vi "SLM Standard Messenger.vi"(0 "Notifier Name":string, 1 "Flat On/Off":bool, 2 "Vortex On/Off":bool, 3 "Top Hat On/Off":bool, 4 "Top Hat Radius":dbl, 5 "Mode Amounts":dbl[](array[numeric]), 6 "Holo Size (px)":i32, 7 "Number of Modes":i32, 8 "SLM Actions":T2, 9 "Holo Position":i32[](array[numeric])) -> (14 "Notifier Name Dup":string, 17 "SLM Status":T1)   [LabVIEW 2018]
uses:
  X10468 Series/X10468 Controls/X10468 SLM Actions.ctl
  X10468 Series/X10468 Controls/X10468 SLM Notifier.ctl
  <vilib>/vision/Image Controls.llb/IMAQ Image.ctl
panel:
  out "Error":errorcluster
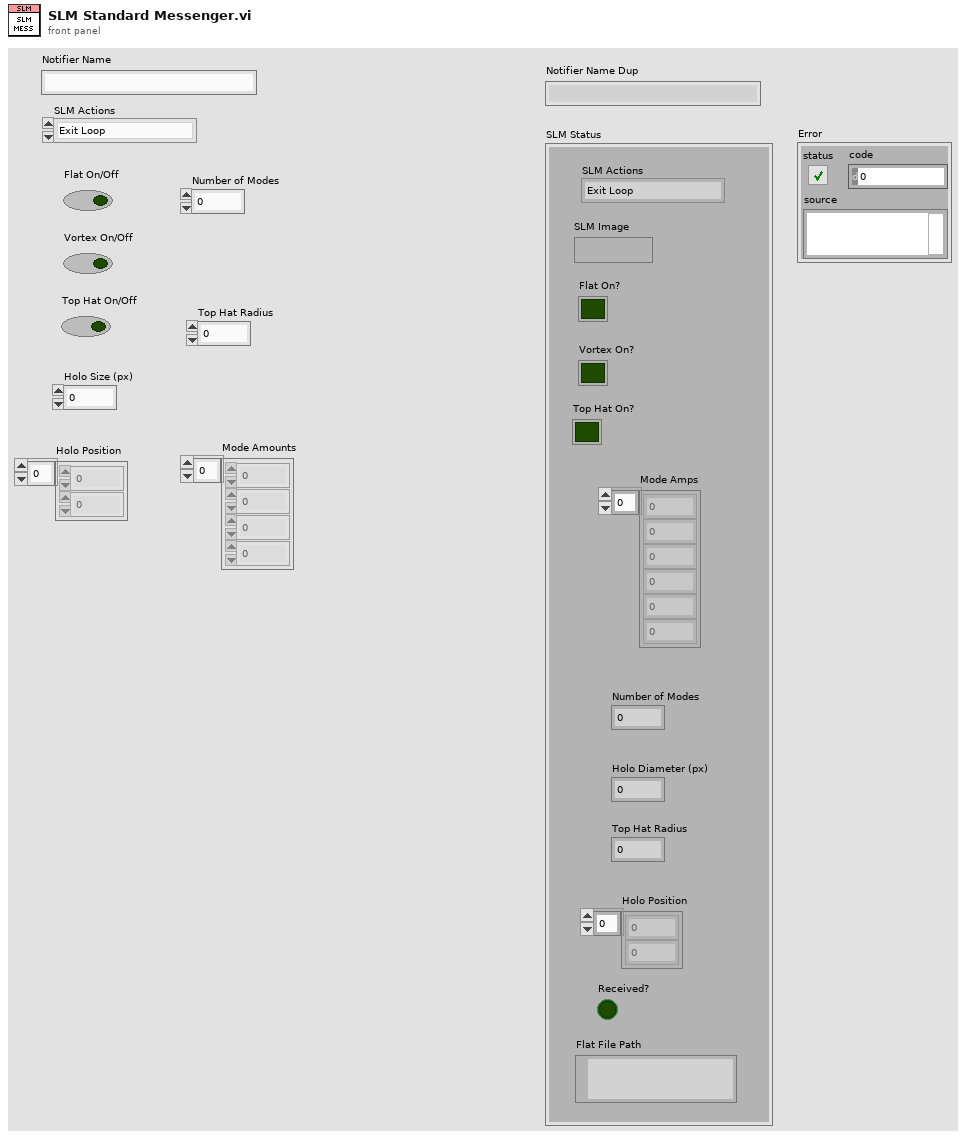
[diagram p1: front panel]
types:
  T1 = typedef "X10468 SLM Notifier.ctl" = cluster{"SLM Actions":T2, "SLM Image":T3, "Flat On?":bool, "Vortex On?":bool, "Top Hat On?":bool, "Mode Amps":dbl[], "Number of Modes":i32, "Holo Diameter (px)":i32, "Top Hat Radius":dbl, "Holo Position":i32[], "Received?":bool, "Flat File Path":path}
  T2 = typedef "X10468 SLM Actions.ctl" = enum16{"Exit Loop", "Get Settings", "Set Flat File", "Change Holo Size", "Change Num Modes", "Change Holo Position", "Change Top Hat Size", "Change Vortex Direction", "Change Mode Amounts", "Flat On/Off", "Vortex On/Off", "Top Hat On/Off", "Make Hologram", "Update SLM Display", "Quit"}
  T3 = typedef "IMAQ Image.ctl" = refnum<image>
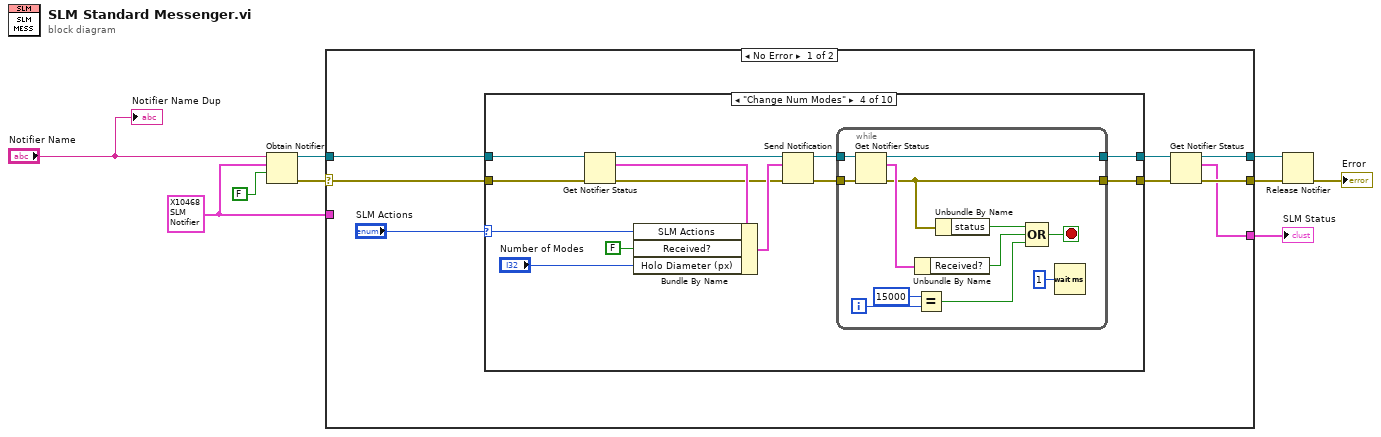
[diagram p0: block diagram]
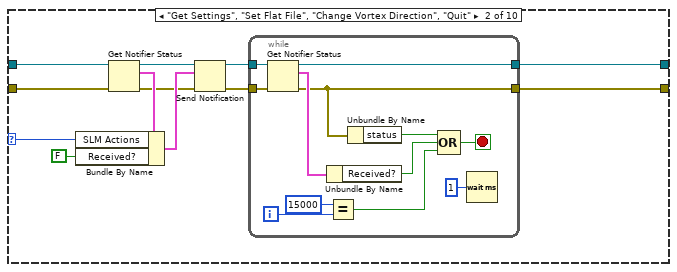
[diagram p3: hidden frame]
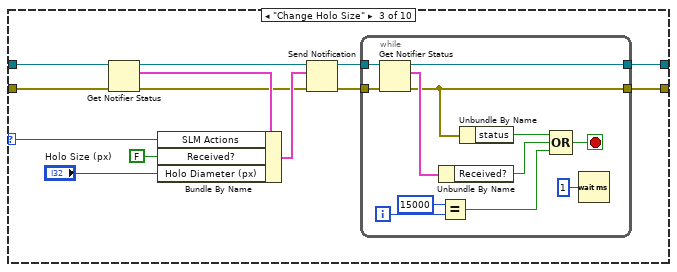
[diagram p4: hidden frame]
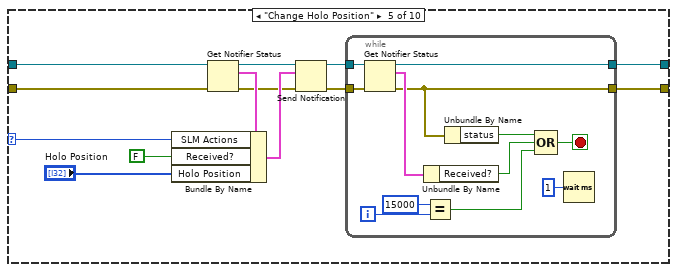
[diagram p5: hidden frame]
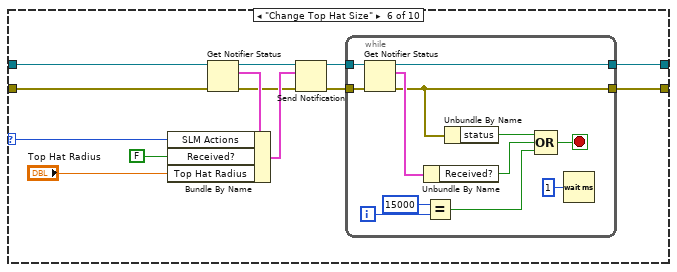
[diagram p6: hidden frame]
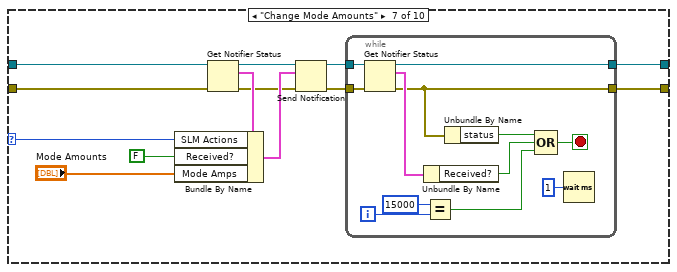
[diagram p7: hidden frame]
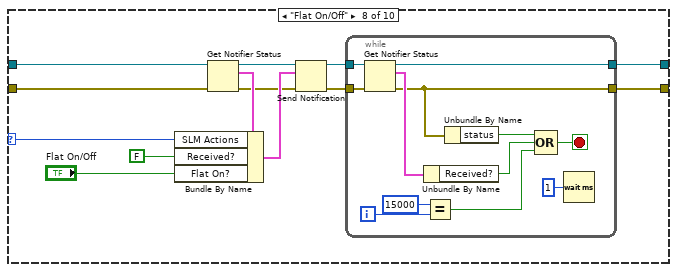
[diagram p8: hidden frame]
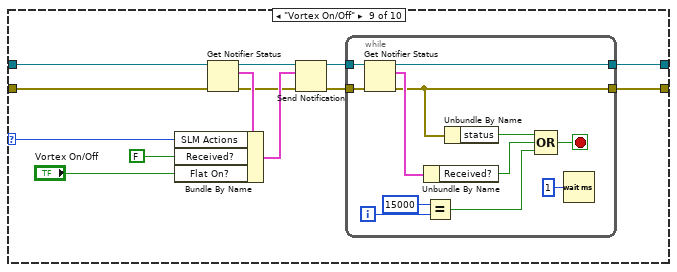
[diagram p9: hidden frame]
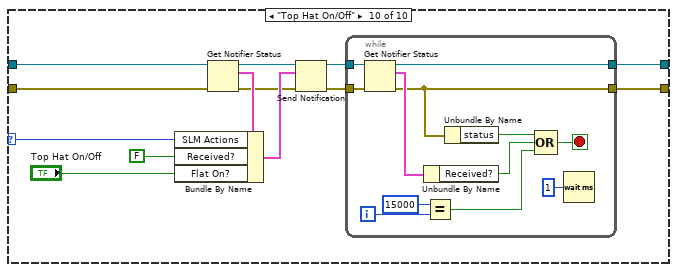
[diagram p10: hidden frame]
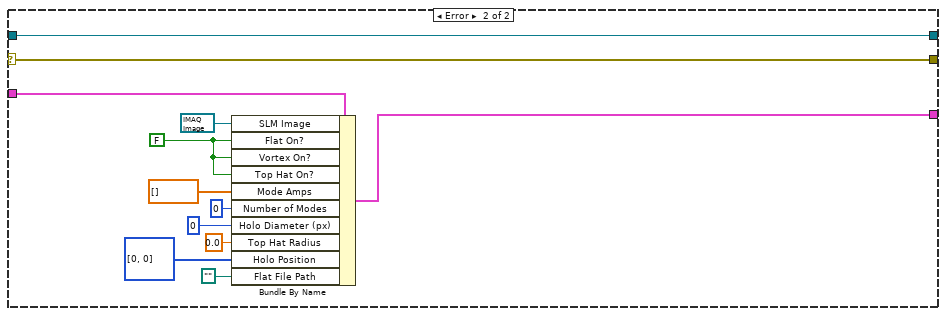
[diagram p11: hidden frame]
diagram:
  w1 = T1 {"SLM Actions"=enum."Exit Loop", "SLM Image"=refnum, "Flat On?"=FALSE, "Vortex On?"=FALSE, "Top Hat On?"=FALSE, "Mode Amps"=[], "Number of Modes"=0, "Holo Diameter (px)"=0, "Top Hat Radius"=0.0, "Holo Position"=[], "Received?"=FALSE, "Flat File Path"=path ""} ("SLM Notifier")
  n1 = Obtain Notifier(name (unnamed)="Notifier Name", notification data type=w1, create if not found? (T)=FALSE) -> (notifier out=w7:refnum<notifier>, error out=w6:errorcluster)  [unwired: 1 in, 1 out]
  n2 = case shown="No Error" w6 {
    selector: w6 -> [w15 w254]
    tunnel: w7 -> [w16 w255]
    tunnel: [w12 w255] -> w5
    tunnel: [w11 w254] -> w4
    tunnel: [w10 w252] -> w2
    tunnel: w1 -> [_ w253]
    frame No Error {
      n3 = case shown="\"Change Num Modes\"" "SLM Actions" {
        selector: "SLM Actions" -> [_ w28 w53 w78 w103 w128 w153 w178 w203 w228]
        tunnel: w16 -> [w19 w31 w56 w81 w106 w131 w156 w181 w206 w231]
        tunnel: w15 -> [w18 w26 w51 w76 w101 w126 w151 w176 w201 w226]
        tunnel: [w19 w21 w46 w71 w96 w121 w146 w171 w196 w221] -> w14
        tunnel: [w18 w20 w45 w70 w95 w120 w145 w170 w195 w220] -> w13
        frame "Exit Loop", Default {
        }
        frame "Get Settings", "Set Flat File", "Change Vortex Direction", "Quit" {
          n4 = Get Notifier Status(notifier=w31, error in (no error)=w26) -> (notifier out=w30:refnum<notifier>, current notification=w29:T1, error out=w25:errorcluster)  [unwired: 2 out]
          n5 = Bundle By Name(cluster=w29, "SLM Actions"=w28, "Received?"=FALSE) -> (w27:T1)
          n6 = Send Notification(notification=w27, notifier=w30, error in (no error)=w25) -> (notifier out=w23:refnum<notifier>, error out=w22:errorcluster)
          n7 = while {
            tunnel: w23 -> [w43]
            tunnel: [w40] -> w21
            tunnel: w22 -> [w37]
            tunnel: [w36] -> w20
            i -> [w39]
            stop <- w32 stop-if-true
            n8 = Get Notifier Status(notifier=w43, error in (no error)=w37) -> (notifier out=w40:refnum<notifier>, current notification=w42:T1, error out=w36:errorcluster)  [unwired: 2 out]
            n9 = Unbundle By Name(w42) -> ("Received?"=w34:bool)
            n10 = Equal?(x=15000, y=w39) -> (x = y?=w33:bool)
            n11 = Unbundle By Name(w36) -> ("status"=w35:bool)
            n12 = Compound Arithmetic op=OR(w35, w34, w33) -> (w32:bool)
            n13 = Wait (ms)(milliseconds to wait=u32 1) -> ()  [unwired: 1 out]
          }
        }
        frame "Change Holo Size" {
          n14 = Get Notifier Status(notifier=w56, error in (no error)=w51) -> (notifier out=w55:refnum<notifier>, current notification=w54:T1, error out=w50:errorcluster)  [unwired: 2 out]
          n15 = Bundle By Name(cluster=w54, "SLM Actions"=w53, "Received?"=FALSE, "Holo Diameter (px)"="Holo Size (px)") -> (w52:T1)
          n16 = Send Notification(notification=w52, notifier=w55, error in (no error)=w50) -> (notifier out=w48:refnum<notifier>, error out=w47:errorcluster)
          n17 = while {
            tunnel: w48 -> [w68]
            tunnel: [w65] -> w46
            tunnel: w47 -> [w62]
            tunnel: [w61] -> w45
            i -> [w64]
            stop <- w57 stop-if-true
            n18 = Get Notifier Status(notifier=w68, error in (no error)=w62) -> (notifier out=w65:refnum<notifier>, current notification=w67:T1, error out=w61:errorcluster)  [unwired: 2 out]
            n19 = Unbundle By Name(w67) -> ("Received?"=w59:bool)
            n20 = Equal?(x=15000, y=w64) -> (x = y?=w58:bool)
            n21 = Unbundle By Name(w61) -> ("status"=w60:bool)
            n22 = Compound Arithmetic op=OR(w60, w59, w58) -> (w57:bool)
            n23 = Wait (ms)(milliseconds to wait=u32 1) -> ()  [unwired: 1 out]
          }
        }
        frame "Change Num Modes" {
          n24 = Get Notifier Status(notifier=w81, error in (no error)=w76) -> (notifier out=w80:refnum<notifier>, current notification=w79:T1, error out=w75:errorcluster)  [unwired: 2 out]
          n25 = Bundle By Name(cluster=w79, "SLM Actions"=w78, "Received?"=FALSE, "Holo Diameter (px)"="Number of Modes") -> (w77:T1)
          n26 = Send Notification(notification=w77, notifier=w80, error in (no error)=w75) -> (notifier out=w73:refnum<notifier>, error out=w72:errorcluster)
          n27 = while {
            tunnel: w73 -> [w93]
            tunnel: [w90] -> w71
            tunnel: w72 -> [w87]
            tunnel: [w86] -> w70
            i -> [w89]
            stop <- w82 stop-if-true
            n28 = Get Notifier Status(notifier=w93, error in (no error)=w87) -> (notifier out=w90:refnum<notifier>, current notification=w92:T1, error out=w86:errorcluster)  [unwired: 2 out]
            n29 = Unbundle By Name(w92) -> ("Received?"=w84:bool)
            n30 = Equal?(x=15000, y=w89) -> (x = y?=w83:bool)
            n31 = Unbundle By Name(w86) -> ("status"=w85:bool)
            n32 = Compound Arithmetic op=OR(w85, w84, w83) -> (w82:bool)
            n33 = Wait (ms)(milliseconds to wait=u32 1) -> ()  [unwired: 1 out]
          }
        }
        frame "Change Holo Position" {
          n34 = Get Notifier Status(notifier=w106, error in (no error)=w101) -> (notifier out=w105:refnum<notifier>, current notification=w104:T1, error out=w100:errorcluster)  [unwired: 2 out]
          n35 = Bundle By Name(cluster=w104, "SLM Actions"=w103, "Received?"=FALSE, "Holo Position"="Holo Position") -> (w102:T1)
          n36 = Send Notification(notification=w102, notifier=w105, error in (no error)=w100) -> (notifier out=w98:refnum<notifier>, error out=w97:errorcluster)
          n37 = while {
            tunnel: w98 -> [w118]
            tunnel: [w115] -> w96
            tunnel: w97 -> [w112]
            tunnel: [w111] -> w95
            i -> [w114]
            stop <- w107 stop-if-true
            n38 = Get Notifier Status(notifier=w118, error in (no error)=w112) -> (notifier out=w115:refnum<notifier>, current notification=w117:T1, error out=w111:errorcluster)  [unwired: 2 out]
            n39 = Unbundle By Name(w117) -> ("Received?"=w109:bool)
            n40 = Equal?(x=15000, y=w114) -> (x = y?=w108:bool)
            n41 = Unbundle By Name(w111) -> ("status"=w110:bool)
            n42 = Compound Arithmetic op=OR(w110, w109, w108) -> (w107:bool)
            n43 = Wait (ms)(milliseconds to wait=u32 1) -> ()  [unwired: 1 out]
          }
        }
        frame "Change Top Hat Size" {
          n44 = Get Notifier Status(notifier=w131, error in (no error)=w126) -> (notifier out=w130:refnum<notifier>, current notification=w129:T1, error out=w125:errorcluster)  [unwired: 2 out]
          n45 = Bundle By Name(cluster=w129, "SLM Actions"=w128, "Received?"=FALSE, "Top Hat Radius"="Top Hat Radius") -> (w127:T1)
          n46 = Send Notification(notification=w127, notifier=w130, error in (no error)=w125) -> (notifier out=w123:refnum<notifier>, error out=w122:errorcluster)
          n47 = while {
            tunnel: w123 -> [w143]
            tunnel: [w140] -> w121
            tunnel: w122 -> [w137]
            tunnel: [w136] -> w120
            i -> [w139]
            stop <- w132 stop-if-true
            n48 = Get Notifier Status(notifier=w143, error in (no error)=w137) -> (notifier out=w140:refnum<notifier>, current notification=w142:T1, error out=w136:errorcluster)  [unwired: 2 out]
            n49 = Unbundle By Name(w142) -> ("Received?"=w134:bool)
            n50 = Equal?(x=15000, y=w139) -> (x = y?=w133:bool)
            n51 = Unbundle By Name(w136) -> ("status"=w135:bool)
            n52 = Compound Arithmetic op=OR(w135, w134, w133) -> (w132:bool)
            n53 = Wait (ms)(milliseconds to wait=u32 1) -> ()  [unwired: 1 out]
          }
        }
        frame "Change Mode Amounts" {
          n54 = Get Notifier Status(notifier=w156, error in (no error)=w151) -> (notifier out=w155:refnum<notifier>, current notification=w154:T1, error out=w150:errorcluster)  [unwired: 2 out]
          n55 = Bundle By Name(cluster=w154, "SLM Actions"=w153, "Received?"=FALSE, "Mode Amps"="Mode Amounts") -> (w152:T1)
          n56 = Send Notification(notification=w152, notifier=w155, error in (no error)=w150) -> (notifier out=w148:refnum<notifier>, error out=w147:errorcluster)
          n57 = while {
            tunnel: w148 -> [w168]
            tunnel: [w165] -> w146
            tunnel: w147 -> [w162]
            tunnel: [w161] -> w145
            i -> [w164]
            stop <- w157 stop-if-true
            n58 = Get Notifier Status(notifier=w168, error in (no error)=w162) -> (notifier out=w165:refnum<notifier>, current notification=w167:T1, error out=w161:errorcluster)  [unwired: 2 out]
            n59 = Unbundle By Name(w167) -> ("Received?"=w159:bool)
            n60 = Equal?(x=15000, y=w164) -> (x = y?=w158:bool)
            n61 = Unbundle By Name(w161) -> ("status"=w160:bool)
            n62 = Compound Arithmetic op=OR(w160, w159, w158) -> (w157:bool)
            n63 = Wait (ms)(milliseconds to wait=u32 1) -> ()  [unwired: 1 out]
          }
        }
        frame "Flat On/Off" {
          n64 = Get Notifier Status(notifier=w181, error in (no error)=w176) -> (notifier out=w180:refnum<notifier>, current notification=w179:T1, error out=w175:errorcluster)  [unwired: 2 out]
          n65 = Bundle By Name(cluster=w179, "SLM Actions"=w178, "Received?"=FALSE, "Flat On?"="Flat On/Off") -> (w177:T1)
          n66 = Send Notification(notification=w177, notifier=w180, error in (no error)=w175) -> (notifier out=w173:refnum<notifier>, error out=w172:errorcluster)
          n67 = while {
            tunnel: w173 -> [w193]
            tunnel: [w190] -> w171
            tunnel: w172 -> [w187]
            tunnel: [w186] -> w170
            i -> [w189]
            stop <- w182 stop-if-true
            n68 = Get Notifier Status(notifier=w193, error in (no error)=w187) -> (notifier out=w190:refnum<notifier>, current notification=w192:T1, error out=w186:errorcluster)  [unwired: 2 out]
            n69 = Unbundle By Name(w192) -> ("Received?"=w184:bool)
            n70 = Equal?(x=15000, y=w189) -> (x = y?=w183:bool)
            n71 = Unbundle By Name(w186) -> ("status"=w185:bool)
            n72 = Compound Arithmetic op=OR(w185, w184, w183) -> (w182:bool)
            n73 = Wait (ms)(milliseconds to wait=u32 1) -> ()  [unwired: 1 out]
          }
        }
        frame "Vortex On/Off" {
          n74 = Get Notifier Status(notifier=w206, error in (no error)=w201) -> (notifier out=w205:refnum<notifier>, current notification=w204:T1, error out=w200:errorcluster)  [unwired: 2 out]
          n75 = Bundle By Name(cluster=w204, "SLM Actions"=w203, "Received?"=FALSE, "Flat On?"="Vortex On/Off") -> (w202:T1)
          n76 = Send Notification(notification=w202, notifier=w205, error in (no error)=w200) -> (notifier out=w198:refnum<notifier>, error out=w197:errorcluster)
          n77 = while {
            tunnel: w198 -> [w218]
            tunnel: [w215] -> w196
            tunnel: w197 -> [w212]
            tunnel: [w211] -> w195
            i -> [w214]
            stop <- w207 stop-if-true
            n78 = Get Notifier Status(notifier=w218, error in (no error)=w212) -> (notifier out=w215:refnum<notifier>, current notification=w217:T1, error out=w211:errorcluster)  [unwired: 2 out]
            n79 = Unbundle By Name(w217) -> ("Received?"=w209:bool)
            n80 = Equal?(x=15000, y=w214) -> (x = y?=w208:bool)
            n81 = Unbundle By Name(w211) -> ("status"=w210:bool)
            n82 = Compound Arithmetic op=OR(w210, w209, w208) -> (w207:bool)
            n83 = Wait (ms)(milliseconds to wait=u32 1) -> ()  [unwired: 1 out]
          }
        }
        frame "Top Hat On/Off" {
          n84 = Get Notifier Status(notifier=w231, error in (no error)=w226) -> (notifier out=w230:refnum<notifier>, current notification=w229:T1, error out=w225:errorcluster)  [unwired: 2 out]
          n85 = Bundle By Name(cluster=w229, "SLM Actions"=w228, "Received?"=FALSE, "Flat On?"="Top Hat On/Off") -> (w227:T1)
          n86 = Send Notification(notification=w227, notifier=w230, error in (no error)=w225) -> (notifier out=w223:refnum<notifier>, error out=w222:errorcluster)
          n87 = while {
            tunnel: w223 -> [w243]
            tunnel: [w240] -> w221
            tunnel: w222 -> [w237]
            tunnel: [w236] -> w220
            i -> [w239]
            stop <- w232 stop-if-true
            n88 = Get Notifier Status(notifier=w243, error in (no error)=w237) -> (notifier out=w240:refnum<notifier>, current notification=w242:T1, error out=w236:errorcluster)  [unwired: 2 out]
            n89 = Unbundle By Name(w242) -> ("Received?"=w234:bool)
            n90 = Equal?(x=15000, y=w239) -> (x = y?=w233:bool)
            n91 = Unbundle By Name(w236) -> ("status"=w235:bool)
            n92 = Compound Arithmetic op=OR(w235, w234, w233) -> (w232:bool)
            n93 = Wait (ms)(milliseconds to wait=u32 1) -> ()  [unwired: 1 out]
          }
        }
      }
      n94 = Get Notifier Status(notifier=w14, error in (no error)=w13) -> (notifier out=w12:refnum<notifier>, current notification=w10:T1, error out=w11:errorcluster)  [unwired: 2 out]
    }
    frame Error {
      w250 = FALSE ("Flat On?")
      n95 = Bundle By Name(cluster=w253, "SLM Image"=T3 refnum, "Flat On?"=w250, "Vortex On?"=w250, "Top Hat On?"=w250, "Mode Amps"=dbl[] [], "Number of Modes"=0, "Holo Diameter (px)"=0, "Top Hat Radius"=0.0, "Holo Position"=i32[] [0, 0], "Flat File Path"=path "") -> (w252:T1)
    }
  }
  "SLM Status" <- w2
  n96 = Release Notifier(notifier=w5, error in (no error)=w4) -> (error out=→"Error":errorcluster)  [unwired: 1 in, 2 out]
  "Notifier Name Dup" <- "Notifier Name"
